vi "Change Bit (U32).vi"(9 "Value":bool=TRUE, 10 "Bit":u8, 11 "Number":u32 format="%.0x") -> (3 "Number Out":u32 format="%.0x")   [LabVIEW 2019, in "Bits.lvlib"]
doc: "Changes a bit in the passed in number to the specified value."
uses:
  Bits.lvlib
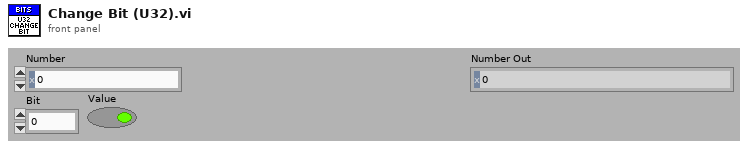
[diagram p1: front panel]
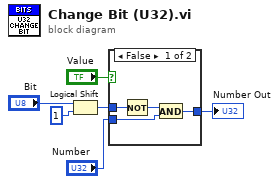
[diagram p0: block diagram]
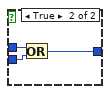
[diagram p2: hidden frame]
diagram:
  n1 = Logical Shift(y="Bit", x=u32 1) -> (x << y=w4:u32)
  n2 = case shown="False" "Value" {
    tunnel: "Number" -> [w9 w13]
    tunnel: [w7 w12] -> w5
    tunnel: w4 -> [w10 w11]
    frame False {
      n3 = Not(x=w10) -> (.not. x?=w8:u32)
      n4 = And(x=w8, y=w9) -> (x .and. y?=w7:u32)
    }
    frame True {
      n5 = Or(x=w11, y=w13) -> (x .or. y?=w12:u32)
    }
  }
  "Number Out" <- w5
